vi "Initialize.vi"(8 "error in (no error)":errorcluster) -> (0 "error out":errorcluster, 3 "AbstractBattery out":refnum<class "AbstractBattery.lvclass">)   [LabVIEW 2011, in "AbstractBattery.lvclass"]
uses:
  AbstractBattery.lvclass
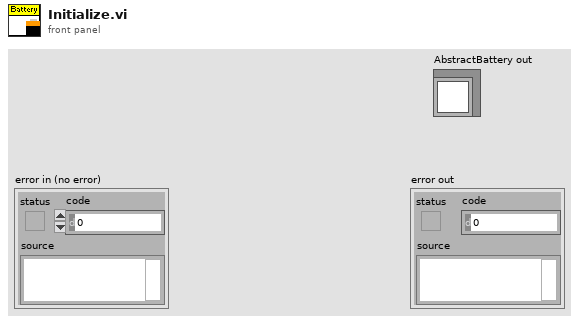
[diagram p1: front panel]
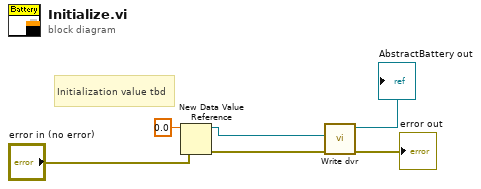
[diagram p0: block diagram]
diagram:
  # "Initialization value tbd"
  n1 = New Data Value Reference(data value=0.0, error in="error in (no error)") -> (data value reference=w3:refnum<data-value>, error out=w5:errorcluster)
  n2 = call "Write dvr.vi"("error in (no error)"=w5, "data value reference"=w3) -> ("error out"=→"error out":errorcluster, "AbstractBattery out"=→"AbstractBattery out":refnum<class "AbstractBattery.lvclass">)  [unwired: 8 in]
